vi "LWXPS_EventExtendedGet.vi"(0 "XPS Reference IN":refnum<k24>, 1 "ID":i32, 5 "LabVIEW error IN":errorcluster) -> (14 "XPS Reference OUT":refnum<k24>, 15 "Returned error code":i32, 16 "Event Trigger Configuration":string, 17 "Action Configuration":string, 18 "XPS Error String":string, 19 "LabVIEW error OUT":errorcluster)   [LabVIEW 2014]
uses:
  D:/XPSQ8_LabView_Library/Development/Source/Dll/Newport.XPS.CommandInterface.dll
  Dll/Newport.XPS.CommandInterface.dll
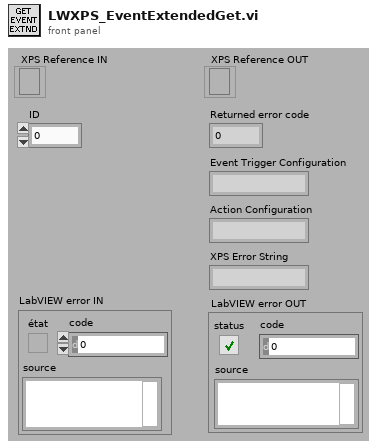
[diagram p1: front panel]
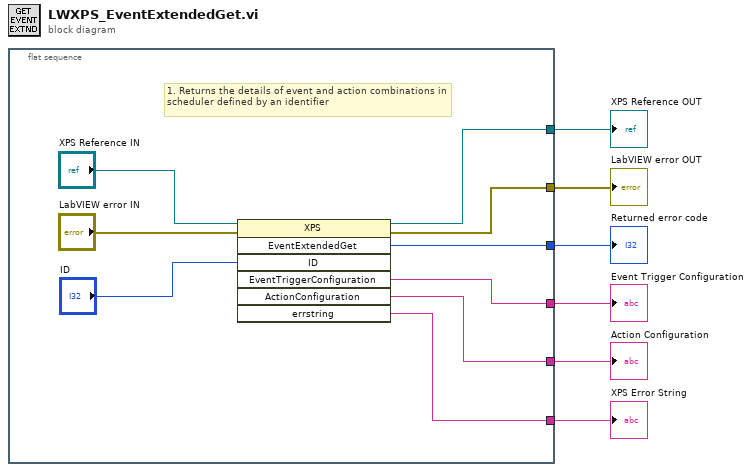
[diagram p0: block diagram]
diagram:
  n1 = flat-sequence {
    tunnel: [w13] -> w6
    tunnel: [w9] -> w5
    tunnel: [w12] -> w4
    tunnel: [w8] -> w3
    tunnel: [w11] -> w2
    tunnel: [w10] -> w1
    frame #0 {
      # "1. Returns the details of event and action combinations in scheduler defined by an identifier"
      n2 = invoke class="XPS" method="EventExtendedGet"(reference="XPS Reference IN", error in="LabVIEW error IN", "ID"="ID") -> (reference out=w13:refnum<k24>, error out=w9:errorcluster, "EventExtendedGet"=w12:i32, "EventTriggerConfiguration"=w8:string, "ActionConfiguration"=w11:string, "errstring"=w10:string)  [unwired: 4 in, 1 out]
    }
  }
  "XPS Reference OUT" <- w6
  "LabVIEW error OUT" <- w5
  "Returned error code" <- w4
  "Event Trigger Configuration" <- w3
  "Action Configuration" <- w2
  "XPS Error String" <- w1
